vi "AttackerBallInGoalieAreaSkill.vi"(6 "AttackerFarback":dbl, 8 "error in (no error)":errorcluster, 9 "Game":refnum<class "Game.lvclass">, 10 "Robot":refnum<class "Robot.lvclass">, 11 "AttackerBallInGoalieAreaSkill in":refnum<class "AttackerBallInGoalieAreaSkill.lvclass">) -> (0 "error out":errorcluster, 2 "Robot out":refnum<class "Robot.lvclass">, 3 "AttackerBallInGoalieAreaSkill out":refnum<class "AttackerBallInGoalieAreaSkill.lvclass">)   [LabVIEW 2018, in "AttackerBallInGoalieAreaSkill.lvclass"]
uses:
  AttackerBallInGoalieAreaSkill.lvclass
  Robot_class/Robot.lvclass
  C:/Users/Gustavo/Desktop/RoboIME/SimplePass/SSL_AI/Object_class/Object.lvclass
  Game_class/Game.lvclass
  Object_class/Object.lvclass/Object.ctl
  Game_class/Game.lvclass/Game.ctl
  Robot_class/Robot.lvclass/Robot.ctl
  Game_class/Read BallRef.vi
  Game_class/Read FieldRef.vi
  Object_class/Read x.vi
  Object_class/Read y.vi
  Robot_class/Write dest_x.vi
  Robot_class/Write dest_y.vi
  Robot_class/Write dest_orientation.vi
  Ball_class/Ball.lvclass
  Field_class/Field.lvclass
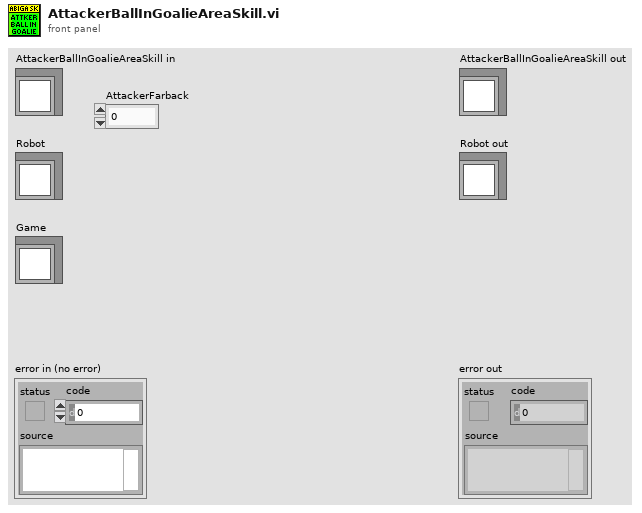
[diagram p1: front panel]
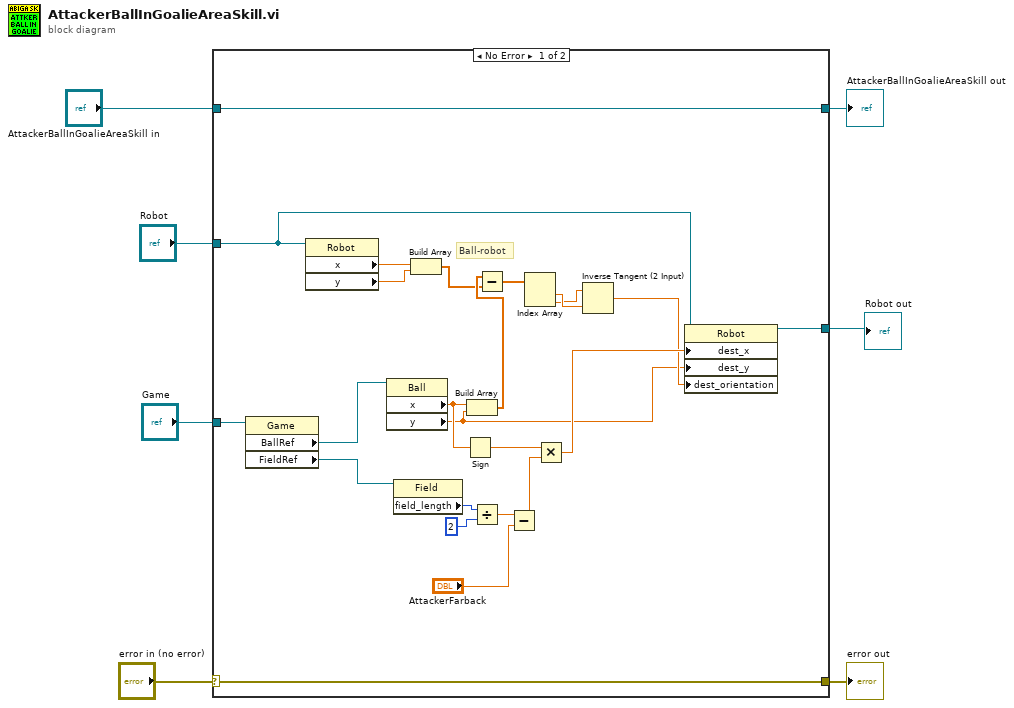
[diagram p0: block diagram]
diagram:
  n1 = case shown="No Error" "error in (no error)" {
    selector: "error in (no error)" -> [w30 w34]
    tunnel: [w30 w34] -> w6
    tunnel: [w31 w33] -> w4
    tunnel: "AttackerBallInGoalieAreaSkill in" -> [w31 w33]
    tunnel: "Robot" -> [w9 w32]
    tunnel: "Game" -> [w27 _]
    tunnel: [w8 w32] -> w1
    frame No Error {
      # "Ball-robot"
      n2 = property class="Game"(reference=w27) -> ("BallRef"=w26:refnum<class "Ball.lvclass">, "FieldRef"=w20:refnum<class "Field.lvclass">)  [unwired: 1 in, 2 out]
      n3 = property class="Robot"(reference=w9) -> ("x"=w29:dbl, "y"=w28:dbl)  [unwired: 1 in, 2 out]
      n4 = property class="Ball"(reference=w26) -> ("x"=w17:dbl, "y"=w10:dbl)  [unwired: 1 in, 2 out]
      n5 = property class="Field"(reference=w20) -> ("field_length"=w19:i32)  [unwired: 1 in, 2 out]
      n6 = Build Array(w29, w28) -> (w24:dbl[])
      n7 = Sign(1:w17) -> (0:w13:dbl)
      n8 = Build Array(w17, w10) -> (w25:dbl[])
      n9 = Divide(x=w19, y=2) -> (x/y=w16:dbl)
      n10 = Subtract(x=w25, y=w24) -> (x-y=w23:dbl[])
      n11 = Subtract(x=w16, y="AttackerFarback") -> (x-y=w14:dbl)
      n12 = Index Array(array=w23) -> (element #1=w22:dbl, element #2=w21:dbl)  [unwired: 2 in]
      n13 = Multiply(x=w13, y=w14) -> (x*y=w12:dbl)
      n14 = Inverse Tangent (2 Input)(1:w22, 2:w21) -> (0:w11:dbl)
      n15 = property class="Robot"(reference=w9, "dest_x"=w12, "dest_y"=w10, "dest_orientation"=w11) -> (reference out=w8:refnum<class "Robot.lvclass">)  [unwired: 1 in, 1 out]
    }
    frame Error {
    }
  }
  "error out" <- w6
  "AttackerBallInGoalieAreaSkill out" <- w4
  "Robot out" <- w1
